vi "ODE Euler Method.vi"(0 "time end":dbl=1.0 format="%.2f", 1 "time start":dbl format="%.2f", 2 "h (step rate)":dbl=0.1 min=0.0 format="%.4f", 3 "X0":dbl[](array[numeric]) format="%.2f", 4 "time":string="t", 5 "X (name of variables)":string[](array[string]), 8 "F(X,t) (right sides of the ODE\nas functions of X and t)":string[](array[string])) -> (6 "Times":dbl[](array[numeric]) format="%.2f", 7 "X Values (solution)":dbl[][](array[numeric]) format="%.2f", 9 "ticks":u32, 10 "error":i32)   [LabVIEW 2020, in "NI_Gmath.lvlib"]
doc: "Solves ordinary differential equations with initial conditions using the Euler method."
uses:
  <vilib>/gmath/NI_Gmath.lvlib
panel:
  out "error message":string
  out "error text":string[](array[string])
  out "error code":i32[](array[numeric])
  # "dX(t)/dt=F(X,t)\nX(0)=X0"
  # "Example:\n\n time start: 0.0 \n time end: 1.0\n h: 0.1\n X0: 1.0 and 1.0 \n time: t\n X: x and y\n F(X,t): sin(t*x)+y and x-y"
  # "further error information"
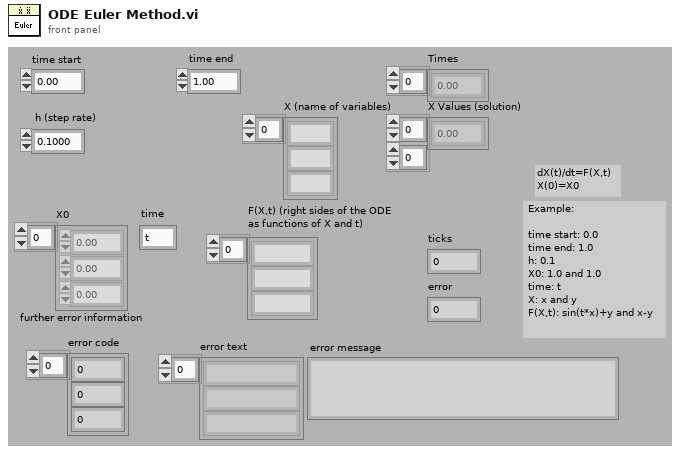
[diagram p1: front panel]
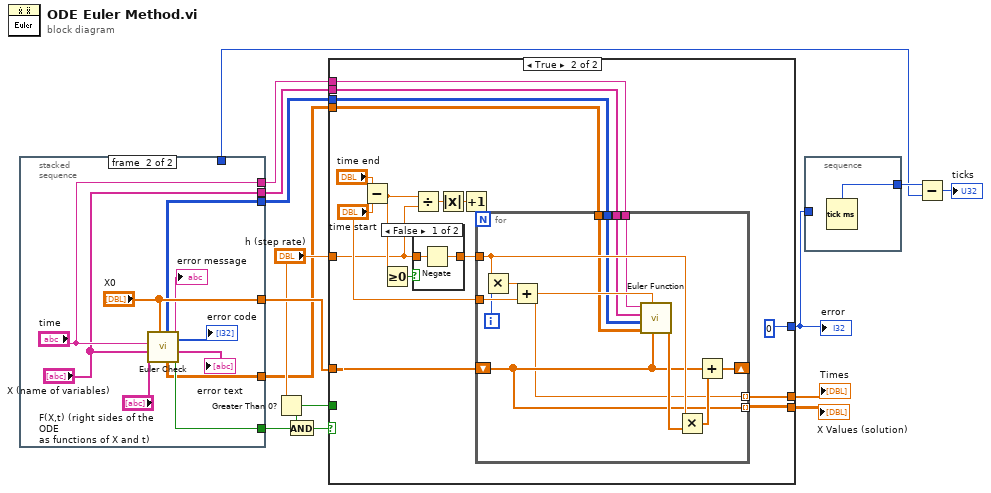
[diagram p0: block diagram]
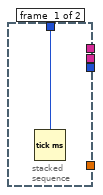
[diagram p2: hidden frame]
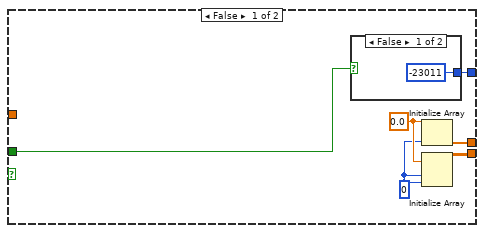
[diagram p3: hidden frame]
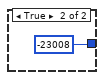
[diagram p4: hidden frame]
diagram:
  n1 = stacked-sequence {
    tunnel: [_ "X0"] -> w13
    tunnel: [_ w25] -> w8
    tunnel: [w16 _] -> w12
    tunnel: [_ "time"] -> w4
    tunnel: [_ "X (name of variables)"] -> w3
    tunnel: [_ w18] -> w2
    tunnel: [_ w17] -> w1
    frame #0 {
      n2 = Tick Count (ms)() -> (millisecond timer value=w16:u32)
    }
    frame #1 {
      n3 = call <vilib>:"Euler Check.vi"("F(X,t)"="F(X,t) (right sides of the ODE\nas functions of X and t)", "X"="X (name of variables)", "time"="time", "X(0)"="X0") -> ("system OK"=w25:bool, "error text"=→"error text":string[], "error"=→"error code":i32[], "error message"=→"error message":string, "result"=w17:dbl[][], "table"=w18:i32[][][])  [unwired: 2 in]
    }
  }
  n4 = Greater Than 0?(x="h (step rate)") -> (x > 0?=w7:bool)
  n5 = And(x=w7, y=w8) -> (x .and. y?=w6:bool)
  n6 = case shown="True" w6 {
    tunnel: [w29 w45] -> w11
    tunnel: [w30 w48] -> w10
    tunnel: w13 -> [_ w47]
    tunnel: [w28 0] -> w5
    tunnel: "h (step rate)" -> [_ w40]
    tunnel: w7 -> [w27 _]
    tunnel: w4 -> [_ w38]
    tunnel: w3 -> [_ w37]
    tunnel: w2 -> [_ w36]
    tunnel: w1 -> [_ w35]
    frame False {
      w31 = 0
      w32 = 0.0
      n7 = case shown="False" w27 {
        tunnel: [-23011 -23008] -> w28
        frame False {
        }
        frame True {
        }
      }
      n8 = Initialize Array(w32, w31) -> (w29:dbl[])
      n9 = Initialize Array(w32, w31, w31) -> (w30:dbl[][])
    }
    frame True {
      n10 = Subtract(x="time end", y="time start") -> (x-y=w42:dbl)
      n11 = Greater Or Equal To 0?(x=w42) -> (x >= 0?=w41:bool)
      n12 = Divide(x=w42, y=w40) -> (x/y=w50:dbl)
      n13 = case shown="False" w41 {
        tunnel: w40 -> [w53 w54]
        tunnel: [w52 w54] -> w39
        frame False {
          n14 = Negate(x=w53) -> (-x=w52:dbl)
        }
        frame True {
        }
      }
      n15 = Absolute Value(x=w50) -> (abs(x)=w43:dbl)
      n16 = Increment(x=w43) -> (x+1=w46:dbl)
      n17 = for {
        N: w46 -> [_]
        shift-right: [w63] -> _
        shift-left: w47 -> [w60]
        tunnel: "time start" -> [w67]
        tunnel: w39 -> [w62]
        tunnel: [w59] -> w45 mode=indexing
        tunnel: [w60] -> w48 mode=indexing
        tunnel: w38 -> [w58]
        tunnel: w37 -> [w57]
        tunnel: w36 -> [w56]
        tunnel: w35 -> [w55]
        i -> [w64]
        n18 = Multiply(x=w62, y=w64) -> (x*y=w65:dbl)
        n19 = Add(x=w65, y=w67) -> (x+y=w59:dbl)
        n20 = call <vilib>:"Euler Function.vi"(6:"X"=w60, 7:"time"=w59, "result"=w55, "table"=w56, 10:"X"=w57, 11:"time"=w58) -> ("F(X,time)"=w61:dbl[])  [unwired: 5 in]
        n21 = Multiply(x=w62, y=w61) -> (x*y=w66:dbl[])
        n22 = Add(x=w60, y=w66) -> (x+y=w63:dbl[])
      }
    }
  }
  "error" <- w5
  "Times" <- w11
  "X Values (solution)" <- w10
  n23 = stacked-sequence {
    tunnel: [w68] -> w15
    tunnel: w5 -> [_]
    frame #0 {
      n24 = Tick Count (ms)() -> (millisecond timer value=w68:u32)
    }
  }
  n25 = Subtract(x=w15, y=w12) -> (x-y=→"ticks":u32)
